vi "UI_Main.vi"() -> ()   [LabVIEW 2024]
uses:
  <vilib>/Utility/file.llb/Write Delimited Spreadsheet (string).vi
panel:
  in  "eXERO":T1(tab)
  out "Sweep Pressure (psig)":dbl
  out "Drycal Flow (sccm)":dbl
  in  "Refresh and Log Frequency (s)":u32=5
  out "Cell Differential":dbl
  out "Exterior (psig)":dbl(knob) scale=0.0..100.0
  out "Interior (psig)":dbl(knob) scale=0.0..100.0
  out "DryCal":dbl(slide) scale=0.0..40.0
  out "MFC_ID":string[](array[string])
  out "Pressure (PSIA)":string[](array[string])
  out "Temperature (C)":string[](array[string])
  out "Volume Flow":string[](array[string])
  out "Mass Flow":string[](array[string])
  out "Set Point":string[](array[string])
  out "Gas":string[](array[string])
  in  "MFC_Data":T2={"MFC_A"={"Setpoint"=0.0, "Units"="SLPM", "MFC_ID"="A", "Full Range"=20.0, "Gas"="Ar"}, "MFC_B"={"Setpoint"=0.0, "Units"="sccm", "MFC_ID"="B", "Full Range"=50.0, "Gas"="H2"}, "MFC_C"={"Setpoint"=0.0, "Units"="sccm", "MFC_ID"="C", "Full Range"=200.0, "Gas"="H2"}, "MFC_D"={"Setpoint"=0.0, "Units"="sccm", "MFC_ID"="D", "Full Range"=200.0, "Gas"="Ar"}, "MFC_E"={"Setpoint"=0.0, "Units"="sccm", "MFC_ID"="E", "Full Range"=100.0, "Gas"="CO2"}, "MFC_E 2"={"Setpoint"=0.0, "Units"="sccm", "MFC_ID"="F", "Full Range"=100.0, "Gas"="CO"}}
  in  "Send MFC Setpoints":bool
  in  "Exterior P Set (0-1000psi)":dbl=1.0
  out "Exterior Set Pressure":dbl
  in  "Exterior P Rate (psi/min)":dbl
  in  "Start Exterior Pressure":bool
  out "Interior (psig)":dbl
  out "Exterior (psig)":dbl
  out "TC1":dbl(slide) scale=0.0..800.0
  out "TC2":dbl(slide) scale=0.0..800.0
  out "TC3":dbl(slide) scale=0.0..800.0
  out "TC4":dbl(slide) scale=0.0..800.0
  in  "Interior P Set (0-500psi)":dbl=1.0
  in  "Interior P Rate (psi/min)":dbl
  in  "Start Interior Pressure":bool
  out "Interior Set Pressure":dbl
  out "Date/Time":string
  in  "EMERGENCY STOP":bool
  out "Exterior Pressure (psig)":dbl
  out "Total Exterior Flow (sccm)":dbl
  out "Interior Pressure (psig)":dbl
  out "Total Interior Flow (sccm)":dbl
  out "TC4":dbl format="%#_2g"
  out "TC3":dbl format="%#_2g"
  out "TC1":dbl format="%#_2g"
  out "TC2":dbl format="%#_2g"
  out "Pressure Differential":cluster{dbl, dbl}(graph) caption="Waveform Chart"
  out "Transducer Median(20) Pressure":T3(graph) caption="Waveform Chart"
  out "Furnace Temperature":cluster{"Median Value":dbl, "Median Value":dbl}(graph) caption="Waveform Chart"
  # "Off"
  # "On"
  # "Off"
  # "On"
  # "Dev Notes"
  # "Takes a second for pressure data to set.\n\nEmergency Shutdown sets all MFCs to 0 and ramps down pressure rapidly (1psi/sec) only if the stop button is pressed. if the stop sign button on top is pressed, test still operates as if nothing was changed."
  # "Chamber Body Temperatures (C)"
  # "TC1"
  # "Interior (not counting VDM)"
  # "TC2"
  # "TC3"
  # "Exterior"
  # "TC4"
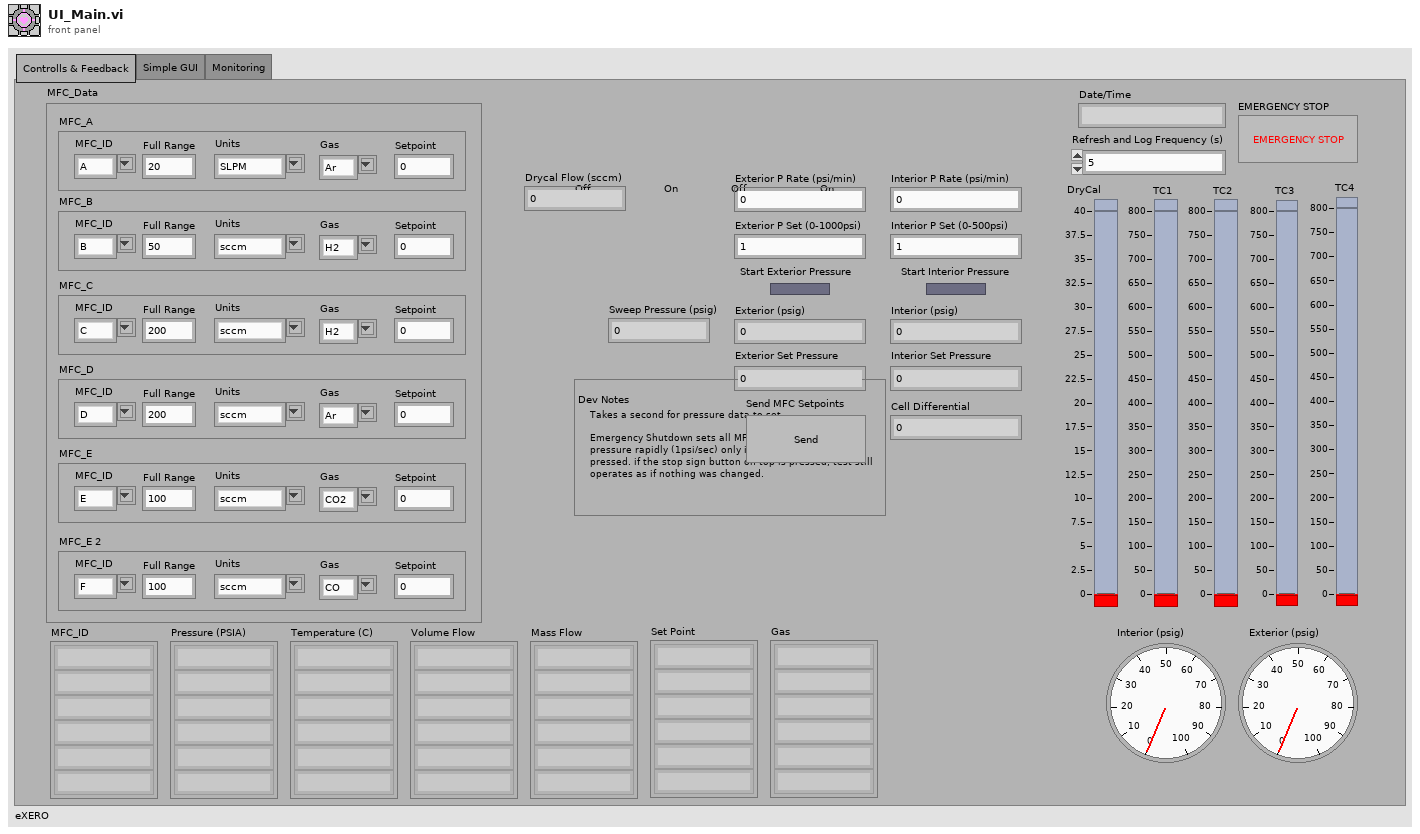
[diagram p1: front panel]
types:
  T1 = enum32{"Controlls & Feedback", "Simple GUI", "Monitoring"}
  T2 = cluster{"MFC_A":cluster{"Setpoint":dbl, "Units":string, "MFC_ID":string, "Full Range":dbl, "Gas":string}, "MFC_B":cluster{"Setpoint":dbl, "Units":string, "MFC_ID":string, "Full Range":dbl, "Gas":string}, "MFC_C":cluster{"Setpoint":dbl, "Units":string, "MFC_ID":string, "Full Range":dbl, "Gas":string}, "MFC_D":cluster{"Setpoint":dbl, "Units":string, "MFC_ID":string, "Full Range":dbl, "Gas":string}, "MFC_E":cluster{"Setpoint":dbl, "Units":string, "MFC_ID":string, "Full Range":dbl, "Gas":string}, "MFC_E 2":cluster{"Setpoint":dbl, "Units":string, "MFC_ID":string, "Full Range":dbl, "Gas":string}}
  T3 = cluster{"[0]":dbl, "[1]":dbl, "[2]":dbl, "[3]":dbl, "[4]":dbl, "[5]":dbl, "[6]":dbl, "[7]":dbl, "[8]":dbl}
  T4 = enum16{"open", "replace", "create", "open or create", "replace or create", "replace or create with confirmation"}
  T5 = cluster{"File Path":path, "error out":errorcluster}
  T6 = cluster{"Setpoint":dbl, "Units":string, "MFC_ID":string, "Full Range":dbl, "Gas":string}[]
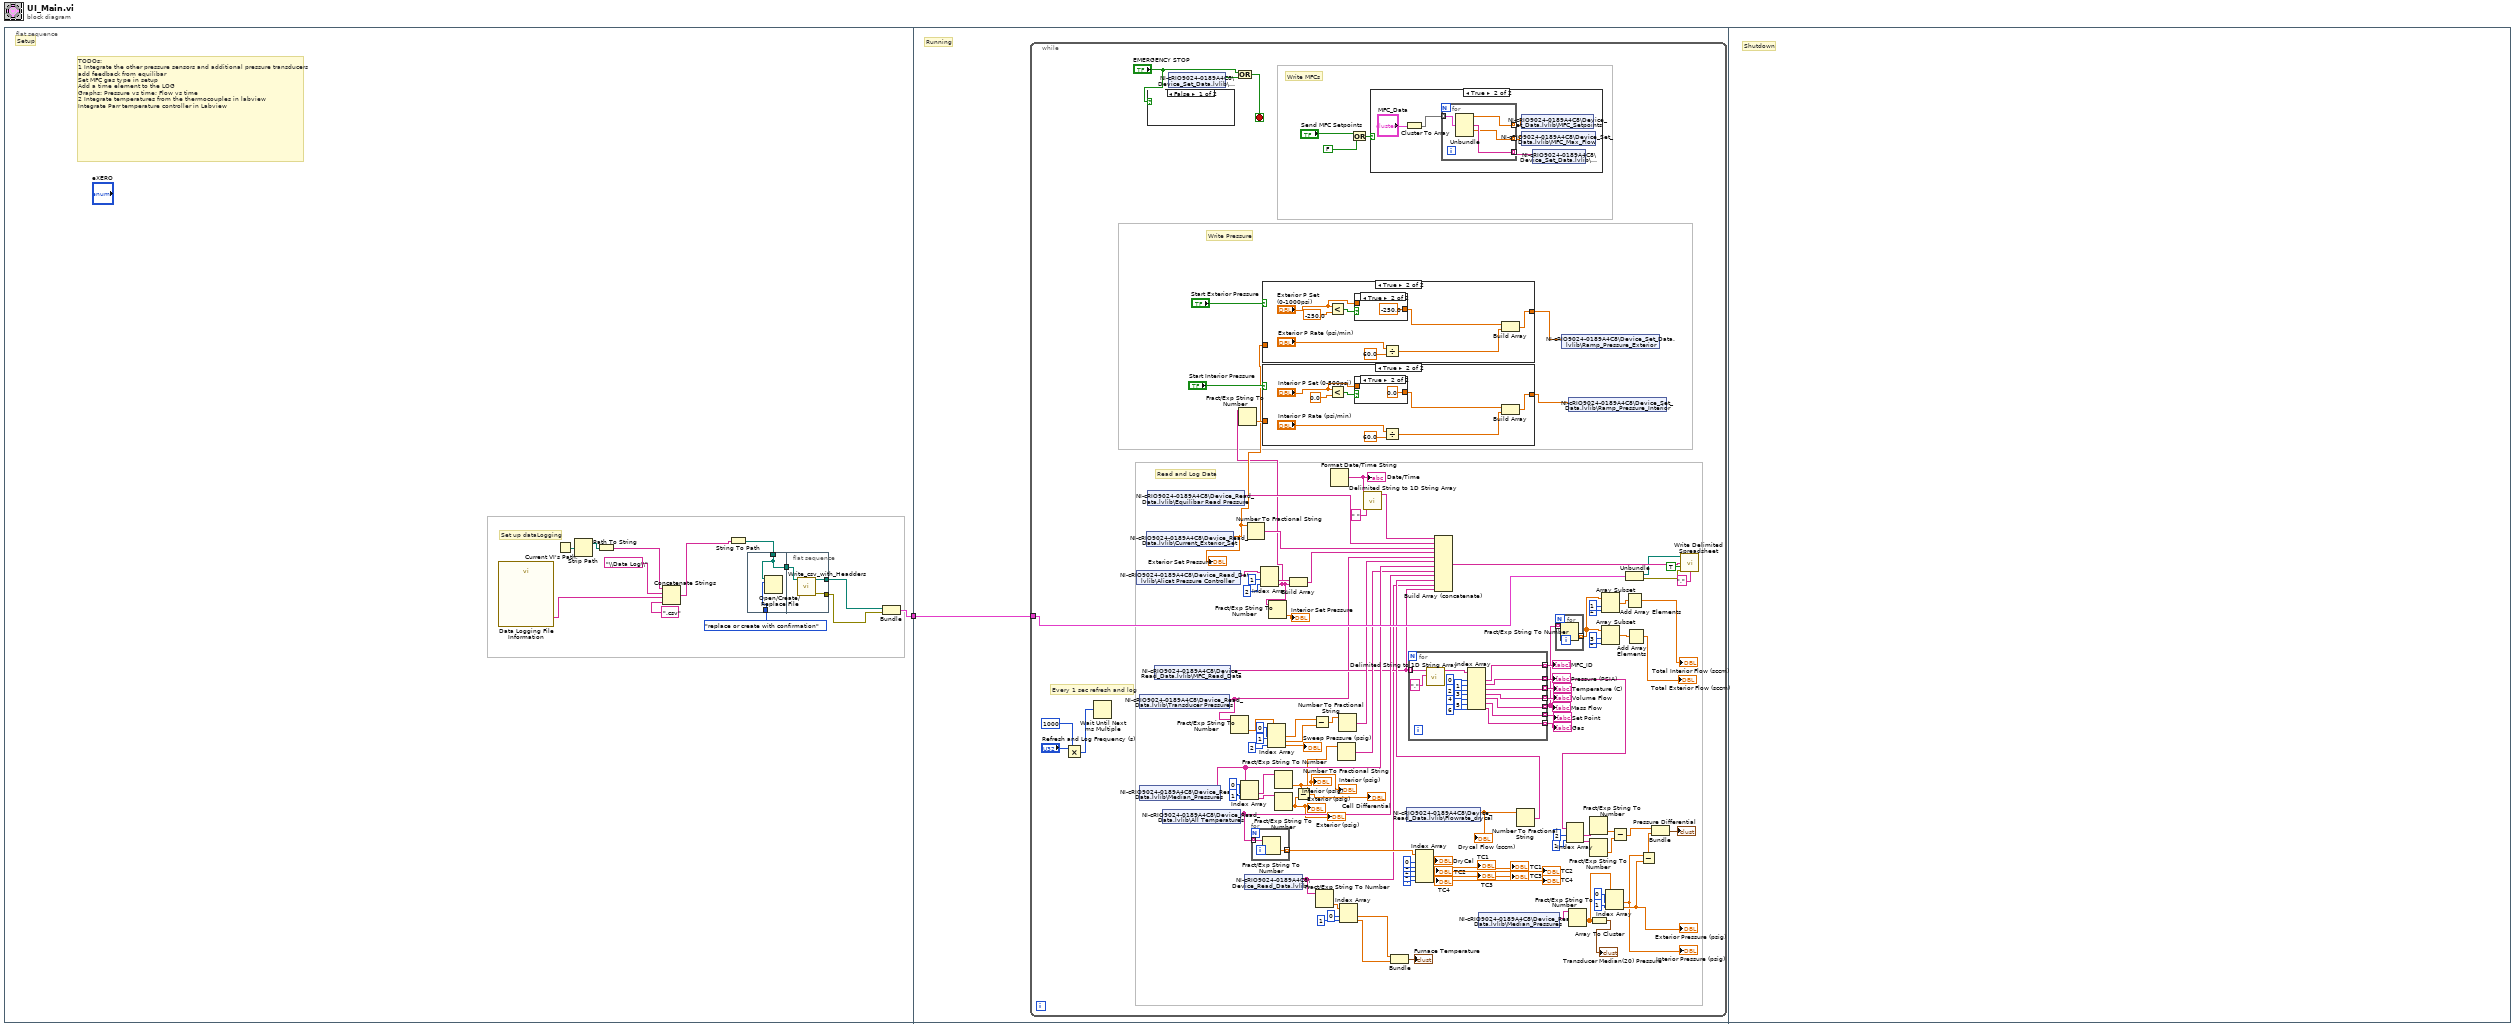
[diagram p0: block diagram]
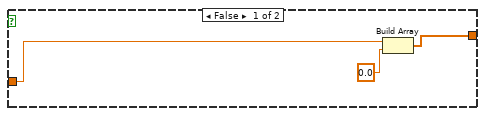
[diagram p2: hidden frame]
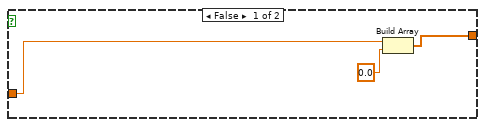
[diagram p4: hidden frame]
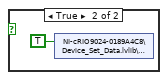
[diagram p6: hidden frame]
diagram:
  n1 = flat-sequence {
    tunnel: [w14] -> w1
    tunnel: w1 -> [w20]
    frame #0 {
      # "TODOs:\n1 Integrate the other pressure sensors and additional pressure transducers\nadd feedback from equilibar\nSet MFC gas type in setup\nAdd a time element to the LOG\nGraphs: Pressure vs time; Flow vs time\n2 Integrate temperatures from the thermocouples in labview\nIntegrate Parr temperature controller in Labview"
      # "Set up dataLogging"
      # "Setup"
      n2 = call "Data Logging File Information"() -> ("File Name"=w2:string)  [unwired: 17 in, 2 out]
      n3 = Current VI's Path() -> (path=w12:path)
      n4 = Strip Path(path=w12) -> (stripped path=w13:path)  [unwired: 1 out]
      n5 = Path To String(path=w13) -> (string=w11:string)
      n6 = Concatenate Strings(w11, "\\Data Log\\", w2, ".csv" ("string")) -> (w3:string)
      n7 = String To Path(string=w3) -> (path=w6:path)
      n8 = flat-sequence {
        tunnel: T4."replace or create with confirmation" ("operation (0:open)") -> [w16]
        tunnel: w6 -> [w15]
        tunnel: [w15] -> w8
        tunnel: [w19] -> w4
        tunnel: [w18] -> w5
        tunnel: w8 -> [w17]
        frame #0 {
          n9 = Open/Create/Replace File(file path (use dialog)=w15, operation (0:open)=w16) -> ()  [unwired: 4 in, 3 out]
        }
        frame #1 {
          n10 = call "Write_csv_with_Headders.vi"("file path (dialog if empty)"=w17) -> ("error out"=w19:errorcluster, "File Path"=w18:path)  [unwired: 9 in]
        }
      }
      n11 = Bundle("File Path"=w5, "error out"=w4) -> (w14:T5)  [unwired: 1 in]
    }
    frame #1 {
      # "Running"
      n12 = while {
        tunnel: w20 -> [w121]
        stop <- w124 stop-if-true
        # "Every 1 sec refresh and log"
        # "Read and Log Data"
        # "Write Pressure"
        # "Write MFCs"
        n13 = Multiply(x="Refresh and Log Frequency (s)", y=u32 1000) -> (x*y=w69:u32)
        n14 = Wait Until Next ms Multiple(millisecond multiple=w69) -> ()  [unwired: 1 out]
        n15 = shared-variable "NI-cRIO9024-0189A4C8\\Device_Read_Data.lvlib\\Alicat Pressure Controller"() -> (w91:string[])  [unwired: 1 in, 1 out]
        n16 = shared-variable "NI-cRIO9024-0189A4C8\\Device_Read_Data.lvlib\\Transducer Pressures"() -> (w33:string[])  [unwired: 1 in, 1 out]
        n17 = shared-variable "NI-cRIO9024-0189A4C8\\Device_Read_Data.lvlib\\Median_Pressures"() -> (w83:string[])  [unwired: 1 in, 1 out]
        n18 = shared-variable "NI-cRIO9024-0189A4C8\\Device_Read_Data.lvlib\\Current_Exterior_Set"() -> (w74:dbl)  [unwired: 1 in, 1 out]
        "Exterior Set Pressure" <- w74
        n19 = case shown="False" "EMERGENCY STOP" {
          frame False {
          }
          frame True {
            n20 = shared-variable "NI-cRIO9024-0189A4C8\\Device_Set_Data.lvlib\\Shutdown"(TRUE ("Shutdown")) -> ()  [unwired: 1 in, 1 out]
          }
        }
        n21 = shared-variable "NI-cRIO9024-0189A4C8\\Device_Read_Data.lvlib\\Equilibar Read Pressure"() -> (w102:string)  [unwired: 1 in, 1 out]
        n22 = shared-variable "NI-cRIO9024-0189A4C8\\Device_Read_Data.lvlib\\MFC_Read_Data"() -> (w43:string[])  [unwired: 1 in, 1 out]
        n23 = shared-variable "NI-cRIO9024-0189A4C8\\Device_Read_Data.lvlib\\All Temperatures"() -> (w82:string[])  [unwired: 1 in, 1 out]
        n24 = shared-variable "NI-cRIO9024-0189A4C8\\Device_Set_Data.lvlib\\Shutdown"() -> (w126:bool)  [unwired: 1 in, 1 out]
        n25 = Fract/Exp String To Number(string=w33) -> (number=w32:dbl[])  [unwired: 3 in, 1 out]
        n26 = Or(x="EMERGENCY STOP", y=w126) -> (x .or. y?=w124:bool)
        n27 = Index Array(array=w83, index #1=0 ("index"), index #2=1 ("index")) -> (element #1=w85:string, element #2=w84:string)
        n28 = shared-variable "NI-cRIO9024-0189A4C8\\Device_Read_Data.lvlib\\Raspi Data"() -> (w42:string[])  [unwired: 1 in, 1 out]
        n29 = Number To Fractional String(number=w74) -> (F-format string=w120:string)  [unwired: 3 in]
        n30 = for {
          tunnel: w82 -> [w143] mode=indexing
          tunnel: [w142] -> w96 mode=indexing
          n31 = Fract/Exp String To Number(string=w143) -> (number=w142:dbl)  [unwired: 3 in, 1 out]
        }
        n32 = Index Array(array=w91, index #1=1 ("index"), index #2=2 ("length")) -> (element #1=w90:string, element #2=w73:string)
        n33 = Fract/Exp String To Number(string=w73) -> (number=w88:dbl)  [unwired: 3 in, 1 out]
        n34 = case shown="True" "Start Exterior Pressure" {
          tunnel: [w145 w154] -> w113
          tunnel: w74 -> [w144 _]
          frame False {
            n35 = Build Array(w144, 0.0 ("element")) -> (w145:dbl[])
          }
          frame True {
            n36 = Less?(x="Exterior P Set (0-1000psi)", y=-250.0) -> (x < y?=w152:bool)
            n37 = case shown="True" w152 {
              tunnel: "Exterior P Set (0-1000psi)" -> [w155 _]
              tunnel: [w155 -250.0 ("Pressure Set (0-1000psi)")] -> w150
              frame False {
              }
              frame True {
              }
            }
            n38 = Divide(x="Exterior P Rate (psi/min)", y=60.0) -> (x/y=w147:dbl)
            n39 = Build Array(w150, w147) -> (w154:dbl[])
          }
        }
        n40 = case shown="True" "Start Interior Pressure" {
          tunnel: [w130 w139] -> w87
          tunnel: w88 -> [w129 _]
          frame False {
            n41 = Build Array(w129, 0.0 ("element")) -> (w130:dbl[])
          }
          frame True {
            n42 = Less?(x="Interior P Set (0-500psi)", y=0.0) -> (x < y?=w137:bool)
            n43 = case shown="True" w137 {
              tunnel: "Interior P Set (0-500psi)" -> [w140 _]
              tunnel: [w140 0.0 ("Pressure Set (0-1000psi)")] -> w135
              frame False {
              }
              frame True {
              }
            }
            n44 = Divide(x="Interior P Rate (psi/min)", y=60.0) -> (x/y=w132:dbl)
            n45 = Build Array(w135, w132) -> (w139:dbl[])
          }
        }
        n46 = Index Array(array=w32, index #1=0 ("index"), index #2=1 ("index"), index #3=2 ("index")) -> (element #1=w29:dbl, element #2=w28:dbl, element #3=→"Sweep Pressure (psig)":dbl)
        n47 = Fract/Exp String To Number(string=w73) -> (number=→"Interior Set Pressure":dbl)  [unwired: 3 in, 1 out]
        n48 = Fract/Exp String To Number(string=w84) -> (number=w80:dbl)  [unwired: 3 in, 1 out]
        "Exterior (psig)" <- w80
        "Exterior (psig)" <- w80
        n49 = Fract/Exp String To Number(string=w85) -> (number=w81:dbl)  [unwired: 3 in, 1 out]
        "Interior (psig)" <- w81
        "Interior (psig)" <- w81
        n50 = Build Array(w90, w73) -> (w89:string[])
        n51 = Subtract(x=w81, y=w80) -> (x-y=w31:dbl)
        "Cell Differential" <- w31
        n52 = Subtract(x=w29, y=w28) -> (x-y=w76:dbl)
        n53 = Fract/Exp String To Number(string=w42) -> (number=w41:dbl[])  [unwired: 3 in, 1 out]
        n54 = Format Date/Time String() -> (date/time string=w105:string)  [unwired: 3 in]
        "Date/Time" <- w105
        n55 = Number To Fractional String(number=w31) -> (F-format string=w79:string)  [unwired: 3 in]
        n56 = Number To Fractional String(number=w76) -> (F-format string=w75:string)  [unwired: 3 in]
        n57 = Index Array(array=w41, index #1=0 ("index"), index #2=1 ("index")) -> (element #1=w37:dbl, element #2=w36:dbl)
        n58 = Or(x="Send MFC Setpoints", y=FALSE) -> (x .or. y?=w123:bool)
        n59 = call <vilib>:"Delimited String to 1D String Array.vi"("delimiter"=" ", "delimited string"=w105) -> ("string array"=w103:string[])  [unwired: 9 in]
        n60 = case shown="True" w123 {
          frame False {
          }
          frame True {
            n61 = Cluster To Array(cluster="MFC_Data") -> (array=w178:T6)
            n62 = for {
              tunnel: w178 -> [w183] mode=indexing
              tunnel: [w182] -> w176 mode=indexing
              tunnel: [w181] -> w177 mode=indexing
              tunnel: [w180] -> w175 mode=indexing
              n63 = Unbundle(w183) -> ("Setpoint"=w181:dbl, "MFC_ID"=w182:string, "Full Range"=w180:dbl)  [unwired: 2 out]
            }
            n64 = shared-variable "NI-cRIO9024-0189A4C8\\Device_Set_Data.lvlib\\MFC_Max_Flow"(w175) -> ()  [unwired: 1 in, 1 out]
            n65 = shared-variable "NI-cRIO9024-0189A4C8\\Device_Set_Data.lvlib\\MFC_Setpoints"(w177) -> ()  [unwired: 1 in, 1 out]
            n66 = shared-variable "NI-cRIO9024-0189A4C8\\Device_Set_Data.lvlib\\MFC_IDs"(w176) -> ()  [unwired: 1 in, 1 out]
          }
        }
        n67 = Bundle("String"=w37, "String"=w36) -> (→"Furnace Temperature":cluster{"String":dbl, "String":dbl})  [unwired: 1 in]
        n68 = shared-variable "NI-cRIO9024-0189A4C8\\Device_Read_Data.lvlib\\Flowrate_drycal"() -> (w35:dbl)  [unwired: 1 in, 1 out]
        "Drycal Flow (sccm)" <- w35
        n69 = for {
          tunnel: w43 -> [w173] mode=indexing
          tunnel: [w163] -> w94 mode=indexing
          tunnel: [w162] -> w66 mode=indexing
          tunnel: [w161] -> w119 mode=indexing
          tunnel: [w160] -> w118 mode=indexing
          tunnel: [w159] -> w54 mode=indexing
          tunnel: [w158] -> w117 mode=indexing
          tunnel: [w157] -> w116 mode=indexing
          n70 = call <vilib>:"Delimited String to 1D String Array.vi"("delimiter"=",", "delimited string"=w173) -> ("string array"=w164:string[])  [unwired: 9 in]
          n71 = Index Array(array=w164, index #1=0 ("index"), index #2=1 ("index"), index #3=2 ("index"), index #4=3 ("index"), index #5=4 ("index"), index #6=5 ("index"), index #7=6 ("index")) -> (element #1=w163:string, element #2=w162:string, element #3=w161:string, element #4=w160:string, element #5=w159:string, element #6=w158:string, element #7=w157:string)
        }
        "MFC_ID" <- w94
        "Pressure (PSIA)" <- w66
        "Volume Flow" <- w118
        "Mass Flow" <- w54
        "Set Point" <- w117
        "Gas" <- w116
        "Temperature (C)" <- w119
        n72 = Index Array(array=w96, index #1=0 ("index"), index #2=1 ("index"), index #3=2 ("index"), index #4=3 ("index"), index #5=4 ("index")) -> (element #1=→"DryCal":dbl, element #2=→"TC1" →"TC1":dbl, element #3=→"TC2" →"TC2":dbl, element #4=→"TC3" →"TC3":dbl, element #5=→"TC4" →"TC4":dbl)
        n73 = shared-variable "NI-cRIO9024-0189A4C8\\Device_Read_Data.lvlib\\Median_Pressures"() -> (w25:string[])  [unwired: 1 in, 1 out]
        n74 = Number To Fractional String(number=w35) -> (F-format string=w44:string)  [unwired: 3 in]
        n75 = Build Array (concatenate)(w103, w102, w120, w89, w33, w75, w83, w79, w82, w44, w42, w43) -> (w110:string[])
        n76 = for {
          tunnel: w54 -> [w128] mode=indexing
          tunnel: [w127] -> w49 mode=indexing
          n77 = Fract/Exp String To Number(string=w128) -> (number=w127:dbl)  [unwired: 3 in, 1 out]
        }
        n78 = shared-variable "NI-cRIO9024-0189A4C8\\Device_Set_Data.lvlib\\Ramp_Pressure_Exterior"(w113) -> ()  [unwired: 1 in, 1 out]
        n79 = Index Array(array=w66, index #1=2 ("index"), index #2=1 ("index")) -> (element #1=w63:string, element #2=w62:string)
        n80 = shared-variable "NI-cRIO9024-0189A4C8\\Device_Set_Data.lvlib\\Ramp_Pressure_Interior"(w87) -> ()  [unwired: 1 in, 1 out]
        n81 = Fract/Exp String To Number(string=w25) -> (number=w24:dbl[])  [unwired: 3 in, 1 out]
        n82 = Fract/Exp String To Number(string=w62) -> (number=w60:dbl)  [unwired: 3 in, 1 out]
        n83 = Fract/Exp String To Number(string=w63) -> (number=w61:dbl)  [unwired: 3 in, 1 out]
        n84 = Array To Cluster(array=w24) -> (cluster=→"Transducer Median(20) Pressure":T3)
        n85 = Array Subset(array=w49, index=1, length=2) -> (w48:dbl[])
        n86 = Array Subset(array=w49, index=3, length=3) -> (w46:dbl[])
        n87 = Index Array(array=w24, index #1=0 ("index"), index #2=1 ("index")) -> (element #1=w22:dbl, element #2=w23:dbl)
        "Interior Pressure (psig)" <- w22
        "Exterior Pressure (psig)" <- w23
        n88 = Subtract(x=w61, y=w60) -> (x-y=w59:dbl)
        n89 = Unbundle(w121) -> ("File Path"=w109:path, "error out"=w108:errorcluster)
        n90 = Add Array Elements(numeric array=w48) -> (sum=→"Total Interior Flow (sccm)":dbl)
        n91 = Add Array Elements(numeric array=w46) -> (sum=→"Total Exterior Flow (sccm)":dbl)
        n92 = Subtract(x=w22, y=w23) -> (x-y=w68:dbl)
        n93 = Bundle(w59, w68) -> (→"Pressure Differential":cluster{dbl, dbl})  [unwired: 1 in]
        n94 = call-poly <vilib>:"Write Delimited Spreadsheet.vi"("file path (dialog if empty)"=w109, "1D data"=w110, "append to file? (new file:F)"=TRUE, "error in (no error)"=w108, "delimiter (\\t)"="," ("delimiter (\\t)")) -> ()  [unwired: 9 in, 2 out]
      }
    }
    frame #2 {
      # "Shutdown"
    }
  }
